vi "Method.vi"(8 "error in (no error)":errorcluster, 11 "Concrete Class in":refnum<class "Concrete Class.lvclass">) -> (0 "error out":errorcluster, 3 "Concrete Class out":refnum<class "Concrete Class.lvclass">)   [LabVIEW 2021, in "Concrete Class.lvclass"]
uses:
  Concrete Class.lvclass
  Concrete Class.lvclass/Concrete Class.ctl
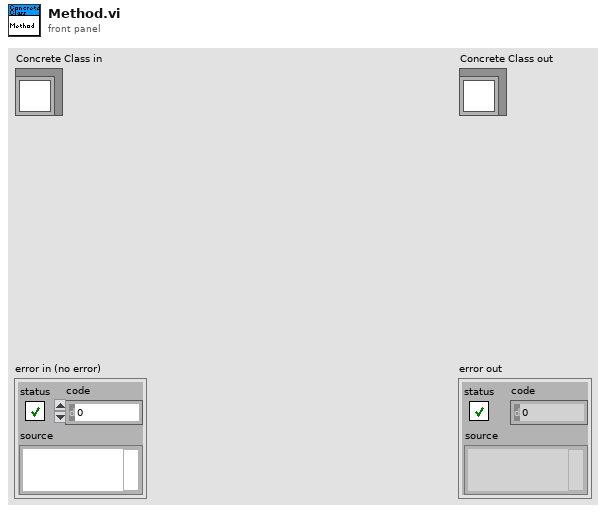
[diagram p1: front panel]
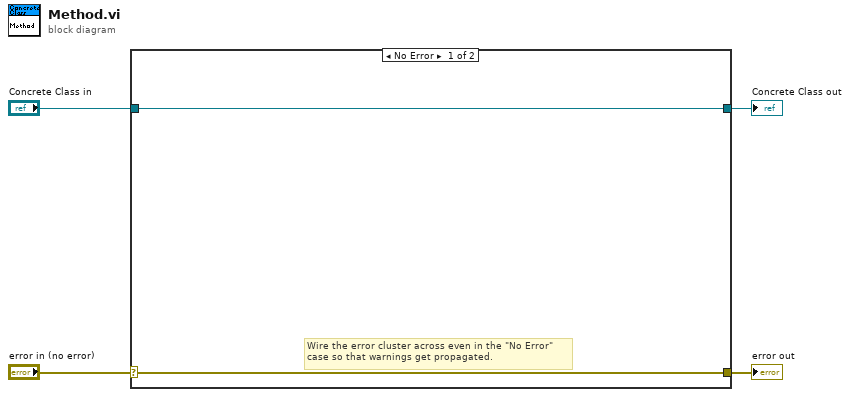
[diagram p0: block diagram]
diagram:
  n1 = case shown="No Error" "error in (no error)" {
    selector: "error in (no error)" -> [w5 w8]
    tunnel: [w5 w8] -> w3
    tunnel: [w6 w7] -> w1
    tunnel: "Concrete Class in" -> [w6 w7]
    frame No Error {
      # "Wire the error cluster across even in the \"No Error\"\ncase so that warnings get propagated."
    }
    frame Error {
    }
  }
  "error out" <- w3
  "Concrete Class out" <- w1
